vi "Generate Documentation--dialog.vi"(8 "error in":errorcluster, 11 "Project Path":path) -> (0 "error out":errorcluster)   [LabVIEW 2019, in "Panther Dashboard.lvlib"]
doc: "<b>Note:</b> This VI was modified by the <b>Validate DQMH Module</b> tool to turn off automatic error handling."
uses:
  Panther Dashboard.lvlib
  <vilib>/Wovalab/AntiDoc/Progress Bar/Progress Bar.lvlib
  <vilib>/Utility/miscctls.llb/LVPointTypeDef.ctl
  <vilib>/Wovalab/AntiDoc/Document Type/Document/Document Type.lvclass
  <vilib>/Wovalab/AntiDoc/Doc/Author Info--cluster.ctl
  <vilib>/Wovalab/AntiDoc/Doc/Doc.lvclass
  <vilib>/Wovalab/AntiDoc/Document Type/Add-ons/LabVIEW Project/Lv Proj/Lv Proj.lvclass
  <vilib>/Wovalab/AntiDoc/Document Type/Add-ons/LabVIEW Project/Lv Proj Config/Lv Proj Config.lvclass
  C:/Program Files (x86)/National Instruments/LabVIEW 2019/vi.lib/Wovalab/AntiDoc/Document Type/Document/Document Type.lvclass
  C:/Program Files (x86)/National Instruments/LabVIEW 2019/vi.lib/Wovalab/AntiDoc/Document Type/Config/Config.lvclass
panel:
  in  "Open the document at the end of the generation":bool=TRUE
  in  "Generate":bool
  out "Progress Bar":u8(slide) caption="Waiting for user action..." max=100 scale=0.0..100.0
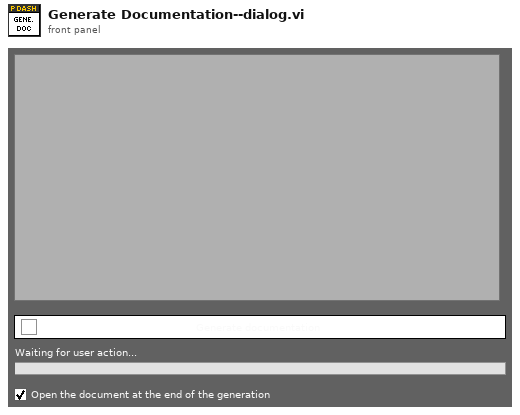
[diagram p1: front panel]
types:
  T1 = enum32{"Invalid", "Standard", "Closed", "Hidden", "Minimized", "Maximized"}
  T2 = typedef "LVPointTypeDef.ctl" = cluster{"Horizontal":i16, "Vertical":i16}
  T3 = typedef "AntiDoc.lvlib/Doc.lvclass/Author Info--cluster.ctl" = cluster{"Name":string, "Email":string}
  T4 = typedef "AntiDoc.lvlib/Document Type.lvclass/Final Documentation Info--cluster.ctl" = cluster{"Title":string, "Author Name":string, "Author Email":string, "Destination Folder":path, "File Name":string}
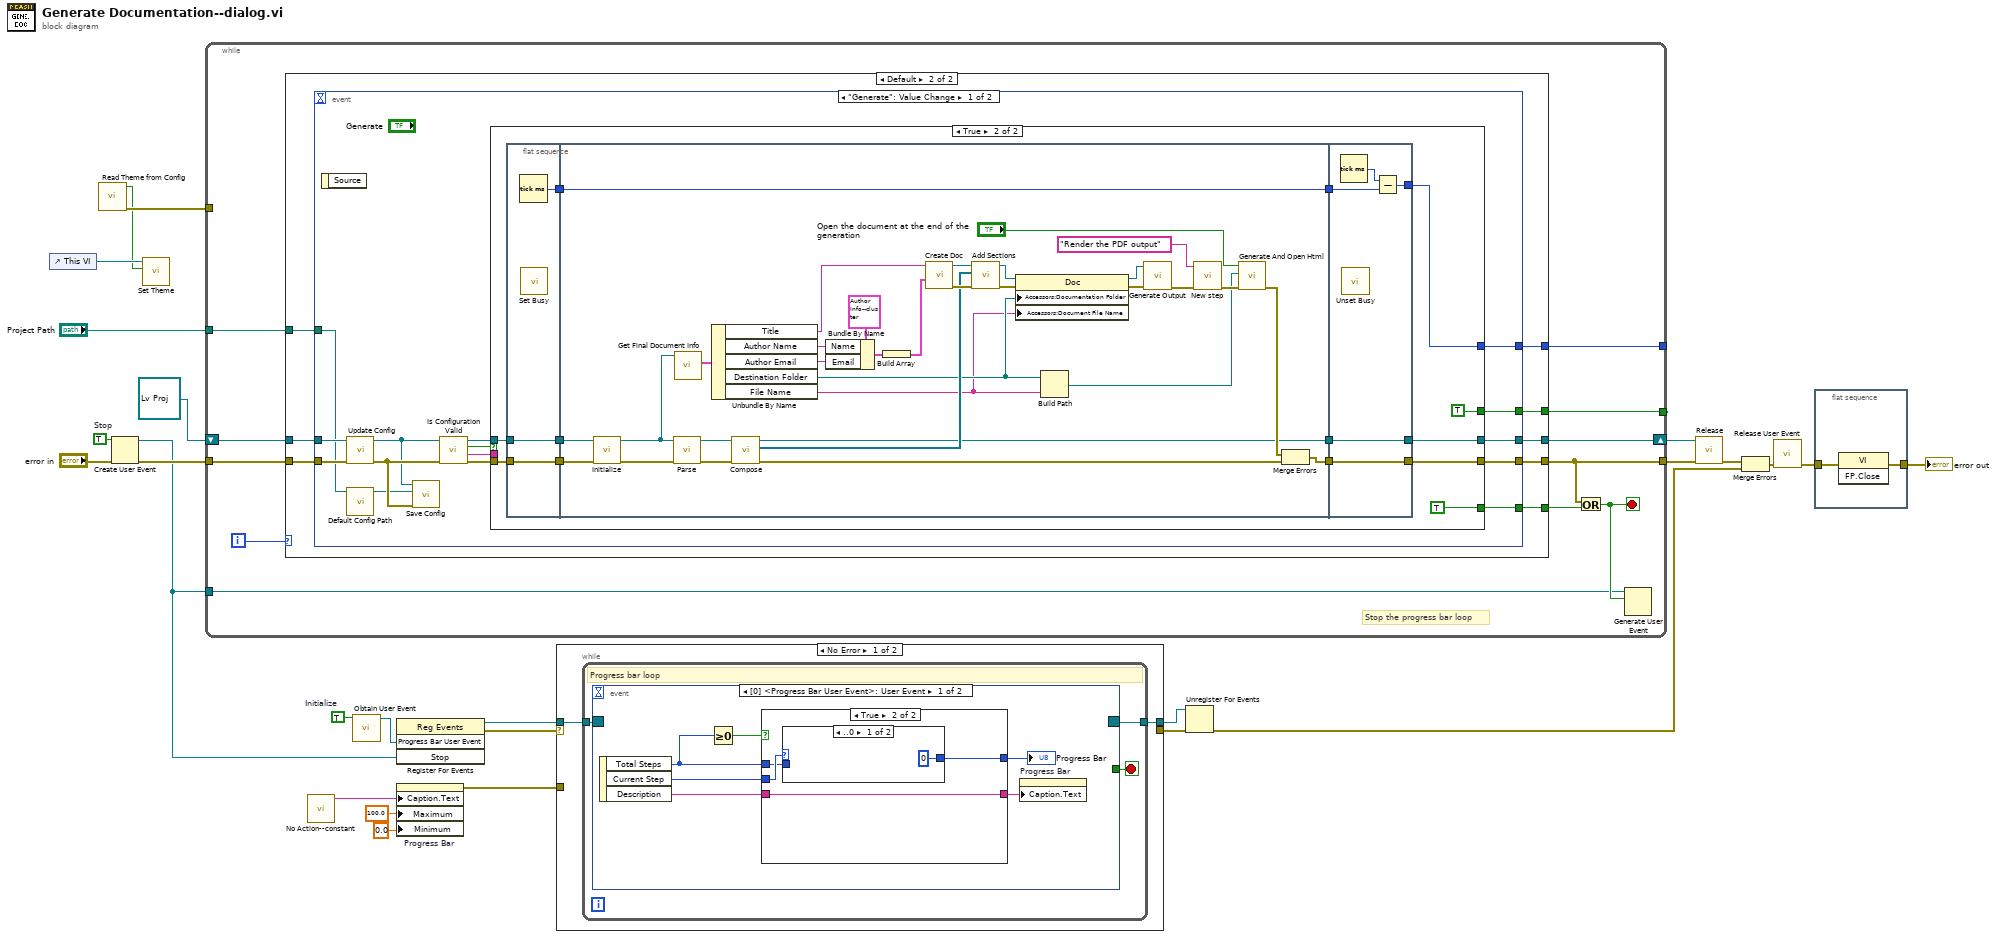
[diagram p0: block diagram]
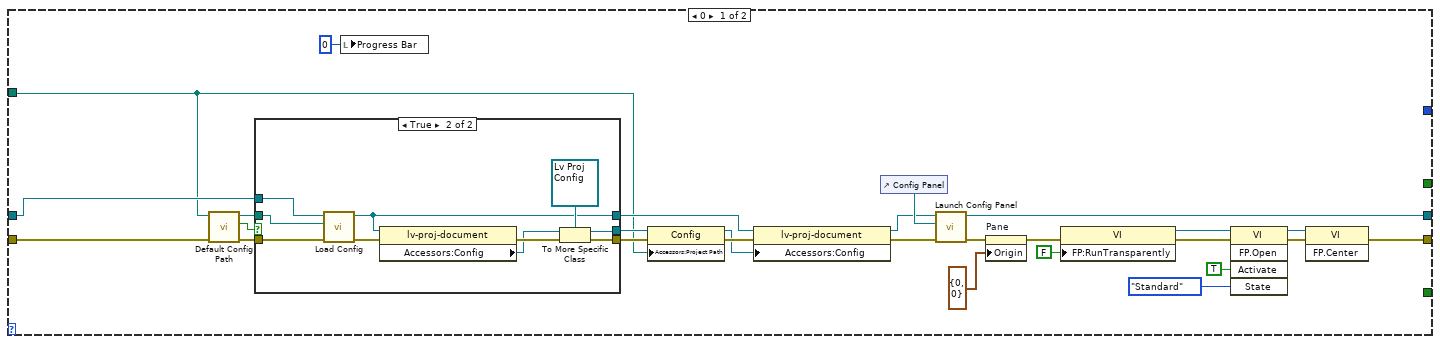
[diagram p2: hidden frame]
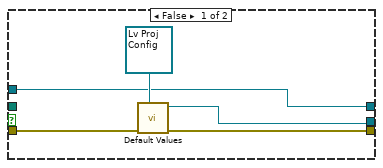
[diagram p3: hidden frame]
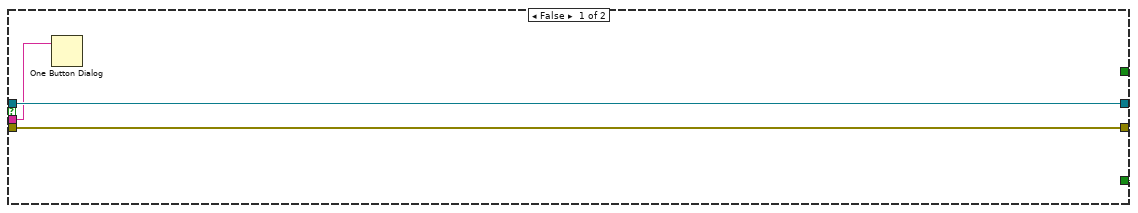
[diagram p4: hidden frame]
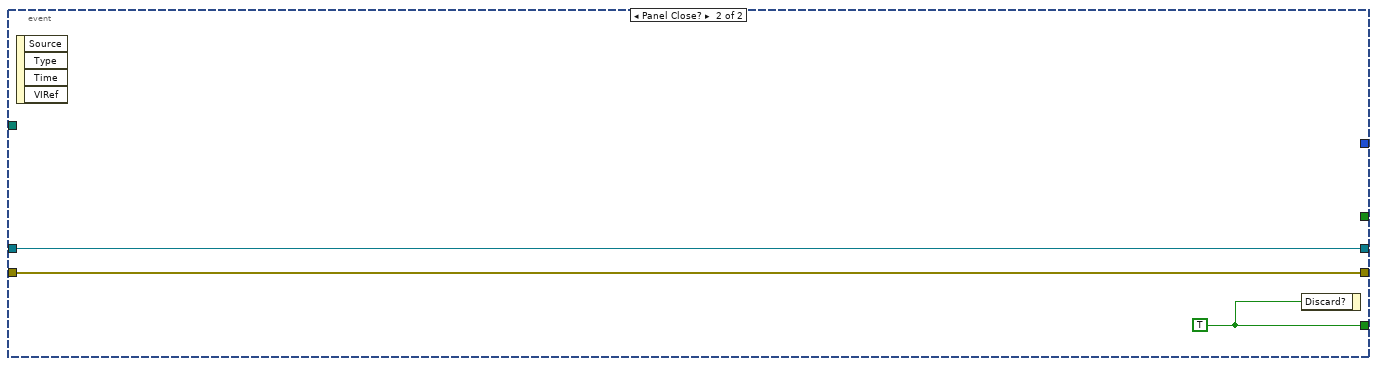
[diagram p5: hidden frame]
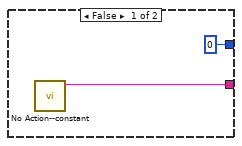
[diagram p6: hidden frame]
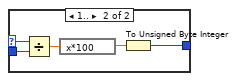
[diagram p7: hidden frame]
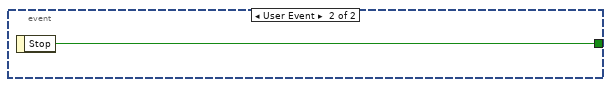
[diagram p8: hidden frame]
diagram:
  w7 = TRUE  # Initialize
  w14 = TRUE  # Stop
  n1 = control-ref of="This VI"() -> (w2:refnum<vi>)
  n2 = call "Read Theme from Config.vi"() -> ("error out"=w15:errorcluster, "Theme"=w1:bool)  [unwired: 10 in]
  n3 = Create User Event(user event datatype=w14, error in="error in") -> (user event=w6:refnum<user-event>, error out=w23:errorcluster)
  n4 = call "Set Theme.vi"("Dark?"=w1, "VI in"=w2) -> ()  [unwired: 10 in]
  n5 = while {
    tunnel: [w36] -> w20
    tunnel: w6 -> [w27]
    tunnel: [w34] -> _
    tunnel: [w33] -> _
    shift-right: [w31] -> w4
    shift-left: refnum<class "Lv Proj.lvclass"> refnum ("Lv Proj Document Type.lvlib:lv-proj-document") -> [w35]
    tunnel: w23 -> [w37]
    tunnel: "Project Path" -> [w28]
    tunnel: w15 -> [_]
    i -> [w32]
    stop <- w30 stop-if-true
    # "Stop the progress bar loop"
    n6 = case shown="Default" w32 {
      tunnel: [w62 w87] -> w36
      tunnel: [_ w85] -> w29
      tunnel: w35 -> [w42 w84]
      tunnel: [_ w83] -> w34
      tunnel: [w47 w82] -> w31
      tunnel: [_ w81] -> w33
      tunnel: w37 -> [w55 w86]
      tunnel: w28 -> [w41 w80]
      frame 0 {
        n7 = call "Default Config Path.vi"("error in"=w55, "Project Path"=w41) -> ("error out"=w56:errorcluster, "File Exists?"=w40:bool, "Config Path"=w39:path)  [unwired: 7 in]
        n8 = case shown="True" w40 {
          tunnel: [w67 w74] -> w46
          tunnel: [w68 w78] -> w59
          tunnel: [w65 w72] -> w43
          tunnel: w42 -> [w65 w71]
          tunnel: w56 -> [w69 w76]
          tunnel: w39 -> [_ w70]
          frame False {
            n9 = call-dynamic "Default Values.vi"("Type"=refnum<class "Lv Proj Config.lvclass"> refnum ("Lv Proj Document Type.lvlib:Config"), "error in"=w69) -> ("error out"=w68:errorcluster, "Config out"=w67:refnum<class "Lv Proj Config.lvclass">)  [unwired: 8 in]
          }
          frame True {
            n10 = call <vilib>:"Load Config.vi"("error in"=w76, "File Path"=w70, "Document in"=w71) -> ("error out"=w77:errorcluster, "Document out"=w72:refnum<class "Lv Proj.lvclass">)  [unwired: 7 in]
            n11 = property class="lv-proj-document"(reference=w72, error in=w77) -> (error out=w79:errorcluster, "Accessors:Config"=w75:refnum<class "Config.lvclass">)  [unwired: 1 out]
            n12 = To More Specific Class(target class=refnum<class "Lv Proj Config.lvclass"> refnum ("Lv Proj Document Type.lvlib:Config"), reference=w75, error in=w79) -> (specific class reference=w74:refnum<class "Lv Proj Config.lvclass">, error out=w78:errorcluster)
          }
        }
        n13 = local write "Progress Bar"(u8 0 ("Progress Bar")) -> ()
        n14 = property class="Config"(reference=w46, error in=w59, "Accessors:Project Path"=w41) -> (reference out=w45:refnum<class "Lv Proj Config.lvclass">, error out=w58:errorcluster)
        n15 = property class="lv-proj-document"(reference=w43, error in=w58, "Accessors:Config"=w45) -> (reference out=w44:refnum<class "Lv Proj.lvclass">, error out=w57:errorcluster)
        n16 = control-ref of="Config Panel"() -> (w48:refnum<vi>)
        n17 = call <vilib>:"Launch Config Panel.vi"("error in"=w57, "Sub Panel"=w48, "Document in"=w44) -> ("error out"=w64:errorcluster, "Document out"=w47:refnum<class "Lv Proj.lvclass">)  [unwired: 7 in]
        n18 = property on="Pane" class="Pane"(error in=w64, "Origin"=T2 {"Horizontal"=0, "Vertical"=0}) -> (error out=w61:errorcluster)  [unwired: 1 in, 1 out]
        n19 = property class="VI"(error in=w61, "FP:RunTransparently"=FALSE ("Front Panel Window:Run VI Transparently")) -> (reference out=w49:refnum<vi>, error out=w60:errorcluster)  [unwired: 1 in]
        n20 = invoke class="VI" method="FP.Open"(reference=w49, error in=w60, "Activate"=TRUE ("Activate?"), "State"=T1."Standard") -> (reference out=w53:refnum<vi>, error out=w63:errorcluster)  [unwired: 1 in, 3 out]
        n21 = invoke class="VI" method="FP.Center"(reference=w53, error in=w63) -> (error out=w62:errorcluster)  [unwired: 1 in, 2 out]
      }
      frame Default {
        n22 = event shown="[0] \"Generate\": Value Change" {
          selector: _ -> [_ _]
          dyn-events: _ -> [_ _]
          timeout: _ -> [_ _]
          tunnel: [w102 w162] -> w87
          tunnel: [w98 w161] -> w85
          tunnel: w84 -> [w94 w160]
          tunnel: [w96 _] -> w83
          tunnel: [w95 w160] -> w82
          tunnel: [w93 _] -> w81
          tunnel: w86 -> [w101 w162]
          tunnel: w80 -> [w89 _]
          event "Generate": Value Change {
            n23 = event-data() -> ()  [unwired: 1 in, 1 out]
            n24 = call <vilib>:"Update Config.vi"("error in"=w101, "Document in"=w94) -> ("error out"=w99:errorcluster, "Document out"=w90:refnum<class "Lv Proj.lvclass">)  [unwired: 8 in]
            n25 = call "Default Config Path.vi"("Project Path"=w89) -> ("Config Path"=w88:path)  [unwired: 8 in, 2 out]
            n26 = call <vilib>:"Save Config.vi"("error in"=w99, "File Path(dialog if empty)"=w88, "Document in"=w90) -> ()  [unwired: 8 in, 1 out]
            n27 = call-dynamic "Is Configuration Valid.vi"("error in"=w99, "Document in"=w90) -> ("error out"=w100:errorcluster, "Details"=w92:string, "Valid?"=w97:bool, "Document out"=w91:refnum<class "Lv Proj.lvclass">)  [unwired: 6 in]
            n28 = case shown="True" w97 {
              tunnel: [w106 w118] -> w102
              tunnel: [FALSE TRUE ("event data")] -> w98
              tunnel: w91 -> [w104 w111]
              tunnel: [_ w110] -> w96
              tunnel: [w104 w108] -> w95
              tunnel: [_ TRUE] -> w93
              tunnel: w92 -> [w103 _]
              tunnel: w100 -> [w106 w116]
              frame False {
                n29 = One Button Dialog(message=w103) -> ()  [unwired: 1 in, 1 out]
              }
              frame True {
                n30 = flat-sequence {
                  tunnel: [w121] -> w113
                  tunnel: [w120] -> w112
                  tunnel: w111 -> [w120]
                  tunnel: [w122] -> w117
                  tunnel: w116 -> [w122]
                  tunnel: [w150] -> w119
                  tunnel: [w137] -> w114
                  tunnel: w113 -> [w137]
                  tunnel: w112 -> [w134]
                  tunnel: w117 -> [w149]
                  tunnel: [w126] -> w107
                  tunnel: [w159] -> w118
                  tunnel: w119 -> [w159]
                  tunnel: w114 -> [w157]
                  tunnel: [w156] -> w110
                  tunnel: [w155] -> w108
                  tunnel: w107 -> [w155]
                  frame #0 {
                    n31 = Tick Count (ms)() -> (millisecond timer value=w121:u32)
                    n32 = call <vilib>:"Set Busy.vi"() -> ()  [unwired: 10 in, 2 out]
                  }
                  frame #1 {
                    n33 = call-dynamic "Initialize.vi"("error in"=w149, "Document in"=w134) -> ("error out"=w148:errorcluster, "Document out"=w133:refnum<class "Lv Proj.lvclass">)  [unwired: 8 in]
                    n34 = call-dynamic "Parse.vi"("error in"=w148, "Document in"=w133) -> ("error out"=w151:errorcluster, "Document out"=w136:refnum<class "Lv Proj.lvclass">)  [unwired: 8 in]
                    n35 = call-dynamic "Get Final Document Info.vi"("Document in"=w133) -> ("Final Documentation Info"=w132:T4)  [unwired: 9 in, 1 out]
                    n36 = Unbundle By Name(w132) -> ("Title"=w131:string, "Author Name"=w130:string, "Author Email"=w129:string, "Destination Folder"=w128:path, "File Name"=w127:string)
                    n37 = call-dynamic "Compose.vi"("error in"=w151, "Document in"=w136) -> ("error out"=w147:errorcluster, "Sections"=w135:refnum<class "Section.lvclass">[], "Document out"=w126:refnum<class "Lv Proj.lvclass">)  [unwired: 7 in]
                    n38 = Bundle By Name(cluster=T3 {"Name"="Wovalab", "Email"="contact@wovalab.com"} ("Author Info"), "Name"=w130, "Email"=w129) -> (w139:T3)
                    n39 = Build Array(w139) -> (w138:T3[])
                    n40 = call <vilib>:"Create Doc.vi"("Authors"=w138, "Title"=w131) -> ("error out"=w154:errorcluster, "Doc out"=w143:refnum<class "Doc.lvclass">)  [unwired: 8 in]
                    n41 = call <vilib>:"Add Sections.vi"("error in (no error)"=w154, "Sections"=w135, "Doc in"=w143) -> ("error out"=w153:errorcluster, "Doc out"=w142:refnum<class "Doc.lvclass">)  [unwired: 7 in]
                    n42 = property class="Doc"(reference=w142, error in=w153, "Accessors:Documentation Folder"=w128, "Accessors:Document File Name"=w127) -> (reference out=w141:refnum<class "Doc.lvclass">, error out=w152:errorcluster)
                    n43 = Build Path(base path=w128, name or relative path=w127) -> (appended path=w125:path)
                    n44 = call <vilib>:"Generate Output.vi"("error in"=w152, "Doc in"=w141) -> ("error out"=w145:errorcluster)  [unwired: 8 in, 1 out]
                    n45 = call <vilib>:"New step.vi"("error in"=w145, "Description"="Render the PDF output") -> ("error out"=w144:errorcluster)  [unwired: 9 in]
                    n46 = call "Generate And Open Html.vi"("error in"=w144, "Generated File Path"=w125, "Open Generated Document"="Open the document at the end of the generation") -> ("error out"=w146:errorcluster)  [unwired: 8 in]
                    n47 = Merge Errors(w146, w147) -> (w150:errorcluster)
                  }
                  frame #2 {
                    n48 = Tick Count (ms)() -> (millisecond timer value=w158:u32)
                    n49 = call <vilib>:"Unset Busy.vi"() -> ()  [unwired: 11 in, 1 out]
                    n50 = Subtract(x=w158, y=w157) -> (x-y=w156:u32)
                  }
                }
              }
            }
          }
          event Panel Close? {
            w161 = TRUE
            n51 = event-data() -> ()  [unwired: 1 in, 4 out]
            n52 = event-data("Discard?"=w161) -> ()  [unwired: 1 in, 1 out]
          }
        }
      }
    }
    n53 = Or(x=w36, y=w29) -> (x .or. y?=w30:bool)
    n54 = Generate User Event(user event=w27, event data cluster=w30) -> ()  [unwired: 2 in, 2 out]
  }
  n55 = call <vilib>:"No Action--constant.vi"() -> ("No Action"=w11:string)  [unwired: 11 in]
  n56 = call <vilib>:"Obtain User Event.vi"("Initialize(F)"=w7) -> ("Progress Bar User Event"=w8:refnum<user-event>)  [unwired: 10 in]
  n57 = register-events(w8, w6) -> (reference out=w9:refnum<event-registration>, error out=w24:errorcluster)  [unwired: 2 in]
  n58 = property on="Progress Bar" class="Slide (strict)"("Caption.Text"=w11, "Maximum"=100.0 ("Data Entry Limits:Maximum"), "Minimum"=0.0 ("Data Entry Limits:Minimum")) -> (error out=w26:errorcluster)  [unwired: 2 in, 1 out]
  n59 = case shown="No Error" w24 {
    selector: w24 -> [_ w188]
    tunnel: w9 -> [w164 w187]
    tunnel: [w163 w187] -> w10
    tunnel: [_ w188] -> w25
    tunnel: w26 -> [_ _]
    frame No Error {
      n60 = while {
        tunnel: w164 -> [w167]
        tunnel: [w165] -> w163
        stop <- w166 stop-if-true
        # "Progress bar loop"
        n61 = event shown="[0] <Progress Bar User Event>: User Event" {
          selector: w167 -> [_ _]
          dyn-events: [_ _] -> w165
          timeout: _ -> [_ _]
          tunnel: [_ w186] -> w166
          event User Event {
            n62 = event-data() -> ("Total Steps"=w170:i32, "Current Step"=w171:i32, "Description"=w172:string)  [unwired: 1 in]
            n63 = Greater Or Equal To 0?(x=w170) -> (x >= 0?=w173:bool)
            n64 = case shown="True" w173 {
              tunnel: w172 -> [_ w176]
              tunnel: w171 -> [_ w179]
              tunnel: w170 -> [_ w178]
              tunnel: [u8 0 w177] -> w169
              tunnel: [w175 w176] -> w168
              frame False {
                n65 = call <vilib>:"No Action--constant.vi"() -> ("No Action"=w175:string)  [unwired: 11 in]
              }
              frame True {
                n66 = case shown="..0" w179 {
                  selector: w179 -> [_ w185]
                  tunnel: w178 -> [_ w184]
                  tunnel: [u8 0 w181] -> w177
                  frame ..0 {
                  }
                  frame 1.. {
                    n67 = Divide(x=w185, y=w184) -> (x/y=w182:dbl)
                    n68 = expression code="x*100"(w182) -> (w183:dbl)
                    n69 = To Unsigned Byte Integer(number=w183) -> (unsigned 8bit integer=w181:u8)
                  }
                }
              }
            }
            "Progress Bar" <- w169
            n70 = property on="Progress Bar" class="Slide (strict)"("Caption.Text"=w168) -> ()  [unwired: 2 in, 2 out]
          }
          event User Event {
            n71 = event-data() -> ("Stop"=w186:bool)  [unwired: 1 in]
          }
        }
      }
    }
    frame Error {
    }
  }
  n72 = Unregister For Events(event registration refnum=w10, error in=w25) -> (error out=w22:errorcluster)
  n73 = call-dynamic "Release.vi"("error in"=w20, "Document in"=w4) -> ("error out"=w19:errorcluster)  [unwired: 9 in]
  n74 = Merge Errors(w19, w22) -> (w21:errorcluster)
  n75 = call <vilib>:"Release User Event.vi"("error in"=w21) -> ("error out"=w18:errorcluster)  [unwired: 10 in]
  n76 = flat-sequence {
    tunnel: w18 -> [w190]
    tunnel: [w189] -> w17
    frame #0 {
      n77 = invoke class="VI" method="FP.Close"(error in=w190) -> (error out=w189:errorcluster)  [unwired: 2 in, 2 out]
    }
  }
  "error out" <- w17
